vi "RT_NetStream.vi"(8 "error in (no error)":errorcluster, 10 "Parameters":T1={"N_Signals_FIFO"=15, "Input Rate (Hz)"=100.0, "Acq Time (s)"=1000.0, "NumOfWarmupIters"=100, "Size fifo"=200, "Period NCL (ms)"=1000, "Timeout fifo Read"=100, "Size Sent Array"=20}, 11 "rt fifo":refnum<k33>) -> (0 "error out":errorcluster)   [LabVIEW 2021]
uses:
  parametersRT.ctl
panel:
  out "element out":dbl[](array[numeric])
  out "Numeric":i32
  out "i":dbl
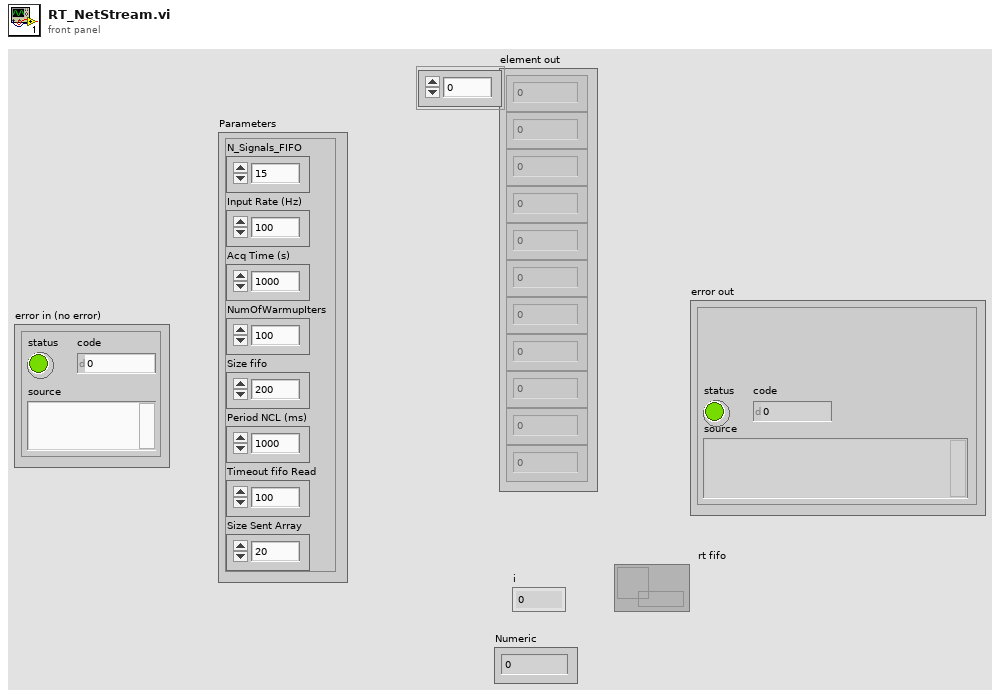
[diagram p1: front panel]
types:
  T1 = typedef "parametersRT.ctl" = cluster{"N_Signals_FIFO":u32, "Input Rate (Hz)":dbl, "Acq Time (s)":dbl, "NumOfWarmupIters":u32, "Size fifo":u32, "Period NCL (ms)":i64, "Timeout fifo Read":i32, "Size Sent Array":i32}
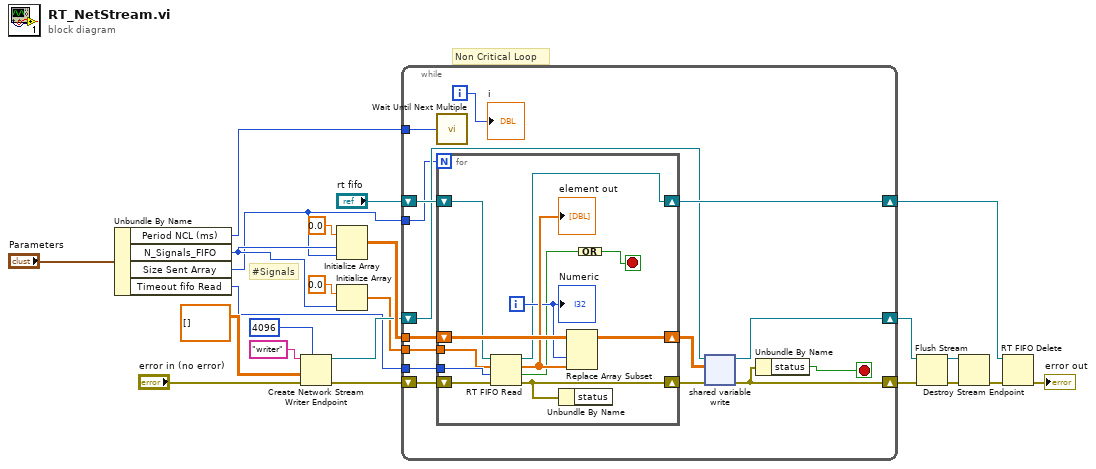
[diagram p0: block diagram]
diagram:
  # "#Signals"
  # "Non Critical Loop"
  n1 = Unbundle By Name("Parameters") -> ("Period NCL (ms)"=w6:i64, "N_Signals_FIFO"=w5:u32, "Size Sent Array"=w4:i32, "Timeout fifo Read"=w3:i32)
  n2 = Create Network Stream Writer Endpoint(7:4096 ("writer buffer size"), 8:"error in (no error)", 9:dbl[][] [], 11:"writer" ("writer name")) -> (0:w2:errorcluster, 3:w8:refnum<k21>)  [unwired: 3 in]
  n3 = Initialize Array(0.0 ("element"), w5, w4) -> (w20:dbl[][])
  n4 = Initialize Array(0.0 ("element"), w5) -> (w7:dbl[])
  n5 = while {
    tunnel: w20 -> [w37]
    tunnel: w4 -> [w29]
    shift-right: [w26] -> w16
    shift-left: w2 -> [w36]
    tunnel: w3 -> [w35]
    shift-right: [w33] -> w13
    shift-left: "rt fifo" -> [w34]
    shift-right: [w32] -> w14
    shift-left: w8 -> [w30]
    tunnel: w7 -> [w28]
    tunnel: w6 -> [w27]
    i -> [w25]
    stop <- w38 stop-if-true
    n6 = call "Wait Until Next Multiple"("Count(mSec)"=w27) -> ()  [unwired: 1 out]
    n7 = for {
      N: w29 -> [_]
      shift-right: [w50] -> w24
      shift-left: w37 -> [w49]
      shift-right: [w41] -> w31
      shift-left: w36 -> [w46]
      tunnel: w35 -> [w45]
      shift-right: [w43] -> w33
      shift-left: w34 -> [w44]
      tunnel: w28 -> [w42]
      i -> [w47]
      stop <- w39 stop-if-true
      n8 = RT FIFO Read(0:w44, 1:w42, 2:w45, 3:w46) -> (8:w43:refnum<k33>, 9:w48:dbl[], 10:w40:bool, 11:w41:errorcluster)  [unwired: 1 out]
      "element out" <- w48
      n9 = Unbundle By Name(w41) -> ()  [unwired: 1 out]
      n10 = Replace Array Subset(array=w49, new element=w48, index (col)=w47) -> (w50:dbl[][])  [unwired: 1 in]
      n11 = Compound Arithmetic op=OR(w40) -> (w39:bool)
      "Numeric" <- w47
    }
    n12 = shared-variable-write(w30, w31, w24) -> (w32:refnum<k21>, w26:errorcluster)  [unwired: 1 in, 1 out]
    n13 = Unbundle By Name(w26) -> ("status"=w38:bool)
    "i" <- w25
  }
  n14 = Flush Stream(8:w16, 11:w14) -> (0:w15:errorcluster, 3:w17:refnum<k21>)  [unwired: 2 in, 1 out]
  n15 = Destroy Stream Endpoint(8:w15, 11:w17) -> (0:w12:errorcluster)
  n16 = RT FIFO Delete(0:w13, 3:w12) -> (11:→"error out":errorcluster)  [unwired: 1 in]
